vi "Enable Panther Logs.vi"() -> ()   [LabVIEW 2016, in "PantherLAB_Log.lvlib"]
uses:
  PantherLAB_Log.lvlib
  <resource>/dialog/lvconfig.llb/LV Config Write Boolean.vi
panel:
  in  "Enable Panther Logs":bool
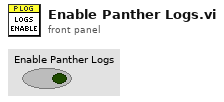
[diagram p1: front panel]
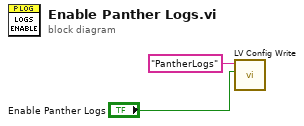
[diagram p0: block diagram]
diagram:
  n1 = call-poly <resource>:"LV Config Write.vi"("value"="Enable Panther Logs", "key"="PantherLogs") -> ()  [unwired: 5 in, 1 out]
